vi "UART_With_Buffer.vi"(0 "COM":refnum<visa-resource-name>, 1 "Timeout (ms)":u32=500, 5 "Function":T1(ring)=enum."SendWaitRead", 7 "Send":string(combo), 9 "Baudrate":u32=115200, 11 "error in (no error)":errorcluster, 12 "Read regular":string="\n") -> (4 "ReceiveString":string, 15 "error out":errorcluster)   [LabVIEW 2020, in "Untitled Library 1.lvlib"]
uses:
  Untitled Library 1.lvlib
  <vilib>/Instr/_visa.llb/VISA Set IO Buffer Mask.ctl
  <vilib>/Instr/_visa.llb/VISA Flush IO Buffer Mask.ctl
  <vilib>/Instr/_visa.llb/VISA Configure Serial Port (Instr).vi
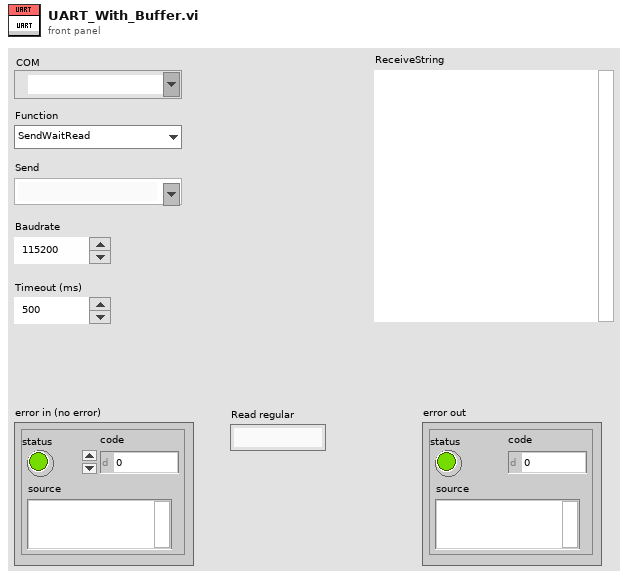
[diagram p1: front panel]
types:
  T1 = enum16{"Open", "Close", "ClearBuffer", "Send", "Read", "SendWaitRead"}
  T2 = enum16{"Open", "Close", "ClearBuffer", "Send", "Read", "SendWaitRead", "SendCompare", "ReadCompare"}
  T3 = typedef "VISA Set IO Buffer Mask.ctl" = u16
  T4 = typedef "VISA Flush IO Buffer Mask.ctl" = u16
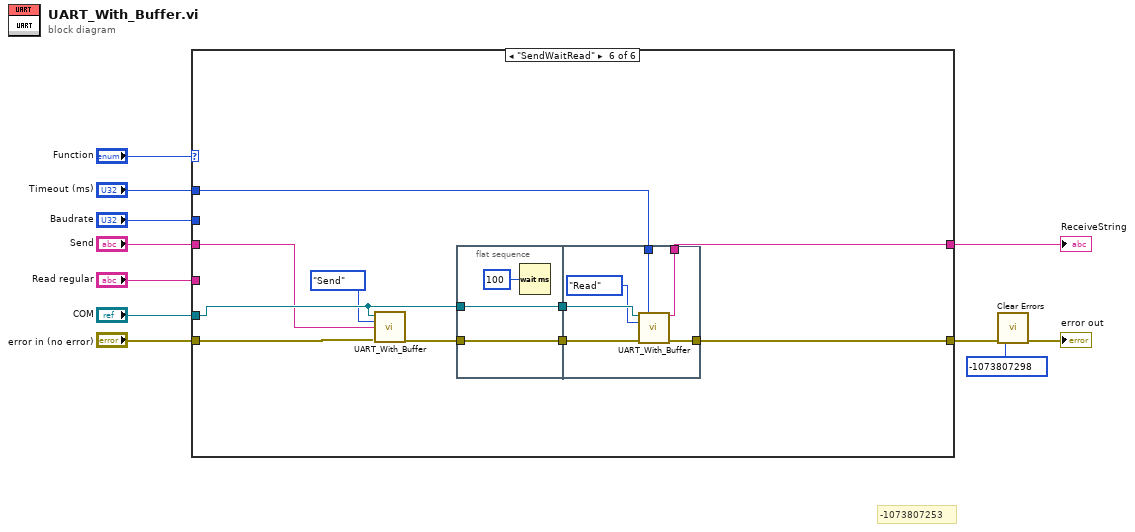
[diagram p0: block diagram]
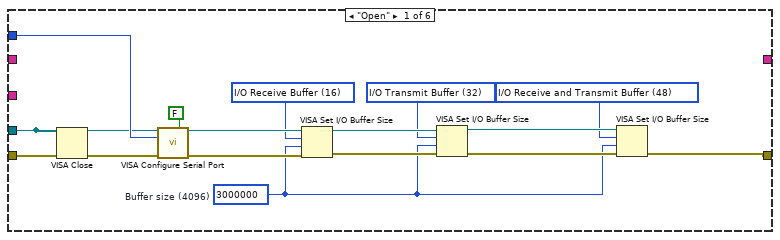
[diagram p2: hidden frame]
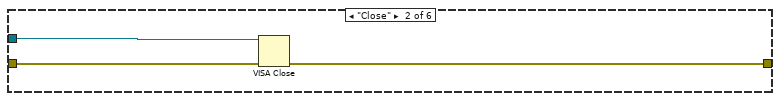
[diagram p3: hidden frame]
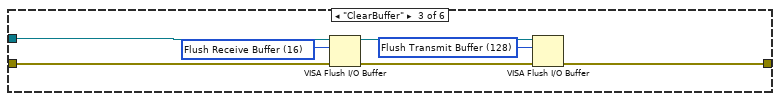
[diagram p4: hidden frame]
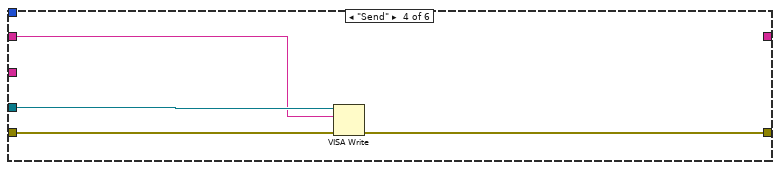
[diagram p5: hidden frame]
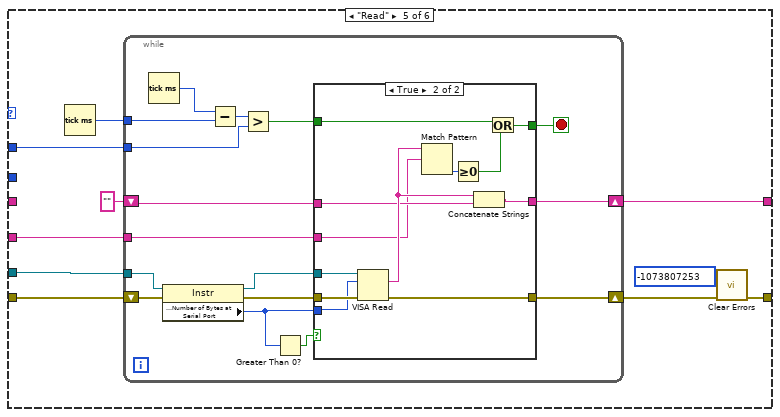
[diagram p6: hidden frame]
diagram:
  # "-1073807253"
  n1 = case shown="\"SendWaitRead\"" "Function" {
    tunnel: "Send" -> [_ _ _ w38 _ w85]
    tunnel: "error in (no error)" -> [w24 w29 w33 w40 w50 w89]
    tunnel: [w12 w28 w36 w41 w46 w92] -> w4
    tunnel: "COM" -> [w25 w30 w32 w39 w51 w90]
    tunnel: "Baudrate" -> [w27 _ _ _ _ _]
    tunnel: "Timeout (ms)" -> [_ _ _ _ w45 w86]
    tunnel: [_ _ _ _ w49 w88] -> w2
    tunnel: "Read regular" -> [_ _ _ _ w42 _]
    frame "Open" {
      w13 = T3 16 items=["I/O Receive Buffer"=16, "I/O Transmit Buffer"=32, "I/O Receive and Transmit Buffer"=48] ("Mask")
      w14 = T3 48 items=["I/O Receive Buffer"=16, "I/O Transmit Buffer"=32, "I/O Receive and Transmit Buffer"=48] ("Mask")
      w15 = T3 32 items=["I/O Receive Buffer"=16, "I/O Transmit Buffer"=32, "I/O Receive and Transmit Buffer"=48] ("Mask")
      w16 = u32 3000000  # Buffer size (4096)
      n2 = VISA Close(VISA resource name=w25, error in (no error)=w24) -> (error out=w23:errorcluster)
      n3 = call-poly "VISA Configure Serial Port"("VISA resource name"=w25, "Enable Termination\nChar (T)"=FALSE ("Enable Termination\nChar (T)"), "baud rate (9600)"=w27, "error in (no error)"=w23) -> ("VISA resource name out"=w21:refnum<visa-resource-name>, "error out"=w22:errorcluster)  [unwired: 4 in, 6 out]
      n4 = VISA Set I/O Buffer Size(VISA resource name=w21, mask (16)=w13, size (4096)=w16, error in (no error)=w22) -> (VISA resource name out=w20:refnum<visa-resource-name>, error out=w18:errorcluster)
      n5 = VISA Set I/O Buffer Size(VISA resource name=w20, mask (16)=w15, size (4096)=w16, error in (no error)=w18) -> (VISA resource name out=w19:refnum<visa-resource-name>, error out=w17:errorcluster)
      n6 = VISA Set I/O Buffer Size(VISA resource name=w19, mask (16)=w14, size (4096)=w16, error in (no error)=w17) -> (error out=w12:errorcluster)  [unwired: 1 out]
    }
    frame "Close" {
      n7 = VISA Close(VISA resource name=w30, error in (no error)=w29) -> (error out=w28:errorcluster)
    }
    frame "ClearBuffer" {
      w35 = T4 16 items=["Flush Receive Buffer"=16, "Write Transmit Buffer to Device"=32, "Flush Receive Buffer (No I/O)"=64, "Flush Transmit Buffer"=128] ("Mask")
      w37 = T4 128 items=["Flush Receive Buffer"=16, "Write Transmit Buffer to Device"=32, "Flush Receive Buffer (No I/O)"=64, "Flush Transmit Buffer"=128] ("Mask")
      n8 = VISA Flush I/O Buffer(VISA resource name=w32, mask (16)=w35, error in (no error)=w33) -> (VISA resource name out=w31:refnum<visa-resource-name>, error out=w34:errorcluster)
      n9 = VISA Flush I/O Buffer(VISA resource name=w31, mask (16)=w37, error in (no error)=w34) -> (error out=w36:errorcluster)  [unwired: 1 out]
    }
    frame "Send" {
      n10 = VISA Write(VISA resource name=w39, write buffer=w38, error in (no error)=w40) -> (error out=w41:errorcluster)  [unwired: 2 out]
    }
    frame "Read" {
      n11 = Tick Count (ms)() -> (millisecond timer value=w44:u32)
      n12 = while {
        tunnel: w51 -> [w67]
        shift-right: [w63] -> w47
        shift-left: w50 -> [w55]
        tunnel: w45 -> [w58]
        tunnel: w44 -> [w60]
        shift-right: [w64] -> w49
        shift-left: "" ("read buffer") -> [w56]
        tunnel: w42 -> [w53]
        stop <- w62 stop-if-true
        n13 = Tick Count (ms)() -> (millisecond timer value=w61:u32)
        n14 = property class="Instr"(reference=w67, error in=w55) -> (reference out=w66:refnum<visa-resource-name>, error out=w54:errorcluster, "Serial Settings:Number of Bytes at Serial Port"=w52:u32)
        n15 = Subtract(x=w61, y=w60) -> (x-y=w59:u32)
        n16 = Greater?(x=w59, y=w58) -> (0:w57:bool)
        n17 = Greater Than 0?(x=w52) -> (x > 0?=w65:bool)
        n18 = case shown="True" w65 {
          tunnel: [w70 w82] -> w63
          tunnel: w54 -> [w70 w81]
          tunnel: w66 -> [_ w80]
          tunnel: [w68 w74] -> w64
          tunnel: w52 -> [_ w72]
          tunnel: [w69 w77] -> w62
          tunnel: w57 -> [w69 w75]
          tunnel: w56 -> [w68 w73]
          tunnel: w53 -> [_ w71]
          frame False {
          }
          frame True {
            n19 = VISA Read(VISA resource name=w80, byte count=w72, error in (no error)=w81) -> (read buffer=w79:string, error out=w82:errorcluster)  [unwired: 2 out]
            n20 = Match Pattern(string=w79, regular expression=w71) -> (offset past match=w78:i32)  [unwired: 1 in, 3 out]
            n21 = Greater Or Equal To 0?(x=w78) -> (x >= 0?=w76:bool)
            n22 = Concatenate Strings(w79, w73) -> (w74:string)
            n23 = Or(x=w75, y=w76) -> (x .or. y?=w77:bool)
          }
        }
      }
      n24 = call <vilib>:"Clear Errors.vi"("error in (no error)"=w47, "specific error code to clear (0: all)"=-1073807253) -> ("error out"=w46:errorcluster)  [unwired: 4 in, 1 out]
    }
    frame "SendWaitRead" {
      n25 = call "UART_With_Buffer.vi"("COM"=w90, "Function"=T2."Send", "Send"=w85, "error in (no error)"=w89) -> ("error out"=w91:errorcluster)  [unwired: 10 in, 1 out]
      n26 = flat-sequence {
        tunnel: w90 -> [w94]
        tunnel: w91 -> [w95]
        tunnel: [w95] -> w84
        tunnel: [w94] -> w83
        tunnel: [w101] -> w92
        tunnel: [w98] -> w88
        tunnel: w86 -> [w97]
        tunnel: w84 -> [w100]
        tunnel: w83 -> [w99]
        frame #0 {
          n27 = Wait (ms)(milliseconds to wait=u32 100) -> ()  [unwired: 1 out]
        }
        frame #1 {
          n28 = call "UART_With_Buffer.vi"("COM"=w99, "Timeout (ms)"=w97, "Function"=T2."Read", "error in (no error)"=w100) -> ("ReceiveString"=w98:string, "error out"=w101:errorcluster)  [unwired: 10 in]
        }
      }
    }
  }
  "ReceiveString" <- w2
  n29 = call <vilib>:"Clear Errors.vi"("error in (no error)"=w4, "specific error code to clear (0: all)"=-1073807298) -> ("error out"=→"error out":errorcluster)  [unwired: 4 in, 1 out]
